vi "FaulhaberV3-Ascii_V1.vi"() -> (1 "searchnames":string[](array[string]), 2 "ID":u32[](array[numeric]), 3 "Faulhaber Objects":T3(array[cluster]))   [LabVIEW 2011] (continued)
actor\" objectType=\"7\" dataType=\"0005\" lowLimit=\"0\" highLimit=\"255\" accessType=\"rw\" defaultValue=\"0\" PDOmapping=\"no\" />\n\t\t\t\t\t<CANopenObject index=\"1010\" name=\"Store parameters\" objectType=\"8\" subNumber=\"10\">\n\t\t\t\t\t\t<CANopenSubObject subIndex=\"00\" name=\"Number of entries\" objectType=\"7\" dataType=\"0005\" accessType=\"ro\" defaultValue=\"9\" PDOmapping=\"no\" objFlags=\"0001\" />\n\t\t\t\t\t\t<CANopenSubObject subIndex=\"01\" name=\"Save all parameters\" objectType=\"7\" dataType=\"0007\" accessType=\"rw\" PDOmapping=\"no\" objFlags=\"0001\" />\n\t\t\t\t\t\t<CANopenSubObject subIndex=\"02\" name=\"Save comm parameters\" objectType=\"7\" dataType=\"0007\" accessType=\"rw\" PDOmapping=\"no\" objFlags=\"0001\" />\n\t\t\t\t\t\t<CANopenSubObject subIndex=\"03\" name=\"Save app parameters\" objectType=\"7\" dataType=\"0007\" accessType=\"rw\" PDOmapping=\"no\" objFlags=\"0001\" />\n\t\t\t\t\t\t<CANopenSubObject subIndex=\"04\" name=\"Save app parameters 1\" objectType=\"7\" dataType=\"0007\" accessType=\"rw\" PDOmapping=\"no\" objFlags=\"0003\" />\n\t\t\t\t\t\t<CANopenSubObject subIndex=\"05\" name=\"Save app parameters 2\" objectType=\"7\" dataType=\"0007\" accessType=\"rw\" PDOmapping=\"no\" objFlags=\"0003\" />\n\t\t\t\t\t\t<CANopenSubObject subIndex=\"06\" name=\"Save cal parameters\" objectType=\"7\" dataType=\"0007\" accessType=\"ro\" PDOmapping=\"no\" objFlags=\"0003\" />\n\t\t\t\t\t\t<CANopenSubObject subIndex=\"07\" name=\"Save factory parameter alls\" objectType=\"7\" dataType=\"0007\" accessType=\"ro\" PDOmapping=\"no\" objFlags=\"0003\" />\n\t\t\t\t\t\t<CANopenSubObject subIndex=\"08\" name=\"Save factory parameters com\" objectType=\"7\" dataType=\"0007\" accessType=\"ro\" PDOmapping=\"no\" objFlags=\"0003\" />\n\t\t\t\t\t\t<CANopenSubObject subIndex=\"09\" name=\"Save factory parameters app\" objectType=\"7\" dataType=\"0007\" accessType=\"ro\" PDOmapping=\"no\" objFlags=\"0003\" />\n\t\t\t\t\t</CANopenObject>\n\t\t\t\t\t<CANopenObject index=\"1011\" name=\"Restore default parameters\" objectType=\"8\" subNumber=\"7\">\n\t\t\t\t\t\t<CANopenSubObject subIndex=\"00\" name=\"Number of entries\" objectType=\"7\" dataType=\"0005\" accessType=\"ro\" defaultValue=\"6\" PDOmapping=\"no\" objFlags=\"0001\" />\n\t\t\t\t\t\t<CANopenSubObject subIndex=\"01\" name=\"Restore all default parameters\" objectType=\"7\" dataType=\"0007\" accessType=\"rw\" PDOmapping=\"no\" objFlags=\"0001\" />\n\t\t\t\t\t\t<CANopenSubObject subIndex=\"02\" name=\"Restore comm default parameters\" objectType=\"7\" dataType=\"0007\" accessType=\"rw\" PDOmapping=\"no\" objFlags=\"0001\" />\n\t\t\t\t\t\t<CANopenSubObject subIndex=\"03\" name=\"Restore app default parameters\" objectType=\"7\" dataType=\"0007\" accessType=\"rw\" PDOmapping=\"no\" objFlags=\"0001\" />\n\t\t\t\t\t\t<CANopenSubObject subIndex=\"04\" name=\"Restore app saved\" objectType=\"7\" dataType=\"0007\" accessType=\"rw\" PDOmapping=\"no\" objFlags=\"0001\" />\n\t\t\t\t\t\t<CANopenSubObject subIndex=\"05\" name=\"Restore app 1 saved\" objectType=\"7\" dataType=\"0007\" accessType=\"rw\" PDOmapping=\"no\" objFlags=\"0001\" />\n\t\t\t\t\t\t<CANopenSubObject subIndex=\"06\" name=\"Restore app 2 saved\" objectType=\"7\" dataType=\"0007\" accessType=\"rw\" PDOmapping=\"no\" objFlags=\"0001\" />\n\t\t\t\t\t</CANopenObject>\n\t\t\t\t\t<CANopenObject index=\"1014\" name=\"COB-ID EMCY\" objectType=\"7\" dataType=\"0007\" accessType=\"rw\" defaultValue=\"$NODEID+0x80\" PDOmapping=\"no\" />\n\t\t\t\t\t<CANopenObject index=\"1016\" name=\"Consumer heartbeat time\" objectType=\"8\" subNumber=\"2\">\n\t\t\t\t\t\t<CANopenSubObject subIndex=\"00\" name=\"Number of entries\" objectType=\"7\" dataType=\"0005\" accessType=\"ro\" defaultValue=\"1\" PDOmapping=\"no\" />\n\t\t\t\t\t\t<CANopenSubObject subIndex=\"01\" name=\"Consumer heartbeat time\" objectType=\"7\" dataType=\"0007\" lowLimit=\"0\" highLimit=\"0x007FFFFF\" accessType=\"rw\" defaultValue=\"0x0\" PDOmapping=\"no\" />\n\t\t\t\t\t</CANopenObject>\n\t\t\t\t\t<CANopenObject index=\"1017\" name=\"Producer heartbeat time\" objectType=\"7\" dataType=\"0006\" lowLimit=\"0\" highLimit=\"65535\" accessType=\"rw\" defaultValue=\"0\" PDOmapping=\"no\" />\n\t\t\t\t\t<CANopenObject index=\"1018\" name=\"Identity object\" objectType=\"9\" subNumber=\"5\">\n\t\t\t\t\t\t<CANopenSubObject subIndex=\"00\" name=\"Number of entries\" objectType=\"7\" dataType=\"0005\" accessType=\"ro\" defaultValue=\"4\" PDOmapping=\"no\" />\n\t\t\t\t\t\t<CANopenSubObject subIndex=\"01\" name=\"Vendor ID\" objectType=\"7\" dataType=\"0007\" accessType=\"ro\" defaultValue=\"327\" PDOmapping=\"no\" />\n\t\t\t\t\t\t<CANopenSubObject subIndex=\"02\" name=\"Product code\" objectType=\"7\" dataType=\"0007\" accessType=\"ro\" PDOmapping=\"no\" />\n\t\t\t\t\t\t<CANopenSubObject subIndex=\"03\" name=\"Revision number\" objectType=\"7\" dataType=\"0007\" lowLimit=\"0x0\" accessType=\"ro\" PDOmapping=\"no\" />\n\t\t\t\t\t\t<CANopenSubObject subIndex=\"04\" name=\"Serial number\" objectType=\"7\" dataType=\"0007\" accessType=\"ro\" PDOmapping=\"no\" />\n\t\t\t\t\t</CANopenObject>\n\t\t\t\t\t<CANopenObject index=\"1029\" name=\"Error behaviour / Number of error classes\" objectType=\"8\" subNumber=\"2\">\n\t\t\t\t\t\t<CANopenSubObject subIndex=\"00\" name=\"Number of error classes\" objectType=\"7\" dataType=\"0005\" accessType=\"ro\" defaultValue=\"1\" PDOmapping=\"no\" />\n\t\t\t\t\t\t<CANopenSubObject subIndex=\"01\" name=\"Communication error\" objectType=\"7\" dataType=\"0005\" PDOmapping=\"no\" uniqueIDRef=\"UID_PARAM_102901\" />\n\t\t\t\t\t</CANopenObject>\n\t\t\t\t\t<CANopenObject index=\"1200\" name=\"Server SDO parameter\" objectType=\"9\" subNumber=\"3\">\n\t\t\t\t\t\t<CANopenSubObject subIndex=\"00\" name=\"Number of entries\" objectType=\"7\" dataType=\"0005\" accessType=\"ro\" defaultValue=\"2\" PDOmapping=\"no\" />\n\t\t\t\t\t\t<CANopenSubObject subIndex=\"01\" name=\"COB-ID client to server (rx)\" objectType=\"7\" dataType=\"0007\" accessType=\"ro\" defaultValue=\"$NODEID+0x600\" PDOmapping=\"no\" />\n\t\t\t\t\t\t<CANopenSubObject subIndex=\"02\" name=\"COB-ID server to client (tx)\" objectType=\"7\" dataType=\"0007\" accessType=\"ro\" defaultValue=\"$NODEID+0x580\" PDOmapping=\"no\" />\n\t\t\t\t\t</CANopenObject>\n\t\t\t\t\t<CANopenObject index=\"1400\" name=\"Receive PDO1 parameter\" objectType=\"9\" subNumber=\"3\">\n\t\t\t\t\t\t<CANopenSubObject subIndex=\"00\" name=\"Number of entries\" objectType=\"7\" dataType=\"0005\" accessType=\"ro\" defaultValue=\"2\" PDOmapping=\"no\" />\n\t\t\t\t\t\t<CANopenSubObject subIndex=\"01\" name=\"COB-ID used by RxPDO1\" objectType=\"7\" dataType=\"0007\" lowLimit=\"1\" highLimit=\"4294967295\" accessType=\"rw\" defaultValue=\"$NODEID+0x200\" PDOmapping=\"no\" />\n\t\t\t\t\t\t<CANopenSubObject subIndex=\"02\" name=\"Transmission type\" objectType=\"7\" dataType=\"0005\" lowLimit=\"0\" highLimit=\"255\" accessType=\"rw\" defaultValue=\"255\" PDOmapping=\"no\" />\n\t\t\t\t\t</CANopenObject>\n\t\t\t\t\t<CANopenObject index=\"1401\" name=\"Receive PDO2 parameter\" objectType=\"9\" subNumber=\"3\">\n\t\t\t\t\t\t<CANopenSubObject subIndex=\"00\" name=\"Number of entries\" objectType=\"7\" dataType=\"0005\" accessType=\"ro\" defaultValue=\"2\" PDOmapping=\"no\" />\n\t\t\t\t\t\t<CANopenSubObject subIndex=\"01\" name=\"COB-ID used by RxPDO2\" objectType=\"7\" dataType=\"0007\" lowLimit=\"1\" highLimit=\"4294967295\" accessType=\"rw\" defaultValue=\"$NODEID+0x300\" PDOmapping=\"no\" />\n\t\t\t\t\t\t<CANopenSubObject subIndex=\"02\" name=\"Transmission type\" objectType=\"7\" dataType=\"0005\" lowLimit=\"0\" highLimit=\"255\" accessType=\"rw\" defaultValue=\"255\" PDOmapping=\"no\" />\n\t\t\t\t\t</CANopenObject>\n\t\t\t\t\t<CANopenObject index=\"1402\" name=\"Receive PDO3 parameters\" objectType=\"9\" subNumber=\"3\">\n\t\t\t\t\t\t<CANopenSubObject subIndex=\"00\" name=\"Number of entries\" objectType=\"7\" dataType=\"0005\" accessType=\"ro\" defaultValue=\"2\" PDOmapping=\"no\" />\n\t\t\t\t\t\t<CANopenSubObject subIndex=\"01\" name=\"COB-ID used by RxPDO3\" objectType=\"7\" dataType=\"0007\" lowLimit=\"1\" highLimit=\"4294967295\" accessType=\"rw\" defaultValue=\"$NODEID+0x400\" PDOmapping=\"no\" />\n\t\t\t\t\t\t<CANopenSubObject subIndex=\"02\" name=\"Transmission type\" objectType=\"7\" dataType=\"0005\" lowLimit=\"0\" highLimit=\"255\" accessType=\"rw\" defaultValue=\"255\" PDOmapping=\"no\" />\n\t\t\t\t\t</CANopenObject>\n\t\t\t\t\t<CANopenObject index=\"1403\" name=\"Receive PDO4 parameter\" objectType=\"9\" subNumber=\"3\">\n\t\t\t\t\t\t<CANopenSubObject subIndex=\"00\" name=\"Number of entries\" objectType=\"7\" dataType=\"0005\" accessType=\"ro\" defaultValue=\"2\" PDOmapping=\"no\" />\n\t\t\t\t\t\t<CANopenSubObject subIndex=\"01\" name=\"COB-ID used by RxPDO4\" objectType=\"7\" dataType=\"0007\" lowLimit=\"1\" highLimit=\"4294967295\" accessType=\"rw\" defaultValue=\"$NODEID+0x500\" PDOmapping=\"no\" />\n\t\t\t\t\t\t<CANopenSubObject subIndex=\"02\" name=\"Transmission type\" objectType=\"7\" dataType=\"0005\" lowLimit=\"0\" highLimit=\"255\" accessType=\"rw\" defaultValue=\"255\" PDOmapping=\"no\" />\n\t\t\t\t\t</CANopenObject>\n\t\t\t\t\t<CANopenObject index=\"1600\" name=\"Receive PDO1 mapping / Number of mapped objects\" objectType=\"9\" subNumber=\"5\">\n\t\t\t\t\t\t<CANopenSubObject subIndex=\"00\" name=\"Number of mapped objects\" objectType=\"7\" dataType=\"0005\" lowLimit=\"0\" highLimit=\"4\" accessType=\"rw\" defaultValue=\"1\" PDOmapping=\"no\" />\n\t\t\t\t\t\t<CANopenSubObject subIndex=\"01\" name=\"RxPDO 1 mapping entry 1\" objectType=\"7\" dataType=\"0007\" lowLimit=\"0\" highLimit=\"4294967295\" accessType=\"rw\" defaultValue=\"0x60400010\" PDOmapping=\"no\" />\n\t\t\t\t\t\t<CANopenSubObject subIndex=\"02\" name=\"RxPDO 1 Mapping entry 2\" objectType=\"7\" dataType=\"0007\" lowLimit=\"0\" highLimit=\"4294967295\" accessType=\"rw\" defaultValue=\"0x0\" PDOmapping=\"no\" />\n\t\t\t\t\t\t<CANopenSubObject subIndex=\"03\" name=\"RxPDO 1 Mapping entry 3\" objectType=\"7\" dataType=\"0007\" lowLimit=\"0\" highLimit=\"4294967295\" accessType=\"rw\" defaultValue=\"0x0\" PDOmapping=\"no\" />\n\t\t\t\t\t\t<CANopenSubObject subIndex=\"04\" name=\"RxPDO 1 Mapping entry 4\" objectType=\"7\" dataType=\"0007\" lowLimit=\"0\" highLimit=\"4294967295\" accessType=\"rw\" defaultValue=\"0x0\" PDOmapping=\"no\" />\n\t\t\t\t\t</CANopenObject>\n\t\t\t\t\t<CANopenObject index=\"1601\" name=\"Receive PDO2 mapping / Number of mapped objects\" objectType=\"9\" subNumber=\"5\">\n\t\t\t\t\t\t<CANopenSubObject subIndex=\"00\" name=\"Number of mapped objects\" objectType=\"7\" dataType=\"0005\" lowLimit=\"0\" highLimit=\"4\" accessType=\"rw\" defaultValue=\"2\" PDOmapping=\"no\" />\n\t\t\t\t\t\t<CANopenSubObject subIndex=\"01\" name=\"RxPDO2 mapping entry 1\" objectType=\"7\" dataType=\"0007\" lowLimit=\"0\" highLimit=\"4294967295\" accessType=\"rw\" defaultValue=\"0x60400010\" PDOmapping=\"no\" />\n\t\t\t\t\t\t<CANopenSubObject subIndex=\"02\" name=\"RxPDO2 mapping entry 2\" objectType=\"7\" dataType=\"0007\" lowLimit=\"0\" highLimit=\"4294967295\" accessType=\"rw\" defaultValue=\"0x607A0020\" PDOmapping=\"no\" />\n\t\t\t\t\t\t<CANopenSubObject subIndex=\"03\" name=\"RxPDO2 mapping entry 3\" objectType=\"7\" dataType=\"0007\" lowLimit=\"0\" highLimit=\"4294967295\" accessType=\"rw\" defaultValue=\"0x0\" PDOmapping=\"no\" />\n\t\t\t\t\t\t<CANopenSubObject subIndex=\"04\" name=\"RxPDO2 mapping entry 4\" objectType=\"7\" dataType=\"0007\" lowLimit=\"0\" highLimit=\"4294967295\" accessType=\"rw\" defaultValue=\"0x0\" PDOmapping=\"no\" />\n\t\t\t\t\t</CANopenObject>\n\t\t\t\t\t<CANopenObject index=\"1602\" name=\"Receive PDO3 mapping / Number of mapped objects\" objectType=\"9\" subNumber=\"5\">\n\t\t\t\t\t\t<CANopenSubObject subIndex=\"00\" name=\"Number of mapped objects\" objectType=\"7\" dataType=\"0005\" lowLimit=\"0\" highLimit=\"4\" accessType=\"rw\" defaultValue=\"2\" PDOmapping=\"no\" />\n\t\t\t\t\t\t<CANopenSubObject subIndex=\"01\" name=\"RxPDO3 mapping entry 1\" objectType=\"7\" dataType=\"0007\" lowLimit=\"0\" highLimit=\"4294967295\" accessType=\"rw\" defaultValue=\"0x60400010\" PDOmapping=\"no\" />\n\t\t\t\t\t\t<CANopenSubObject subIndex=\"02\" name=\"RxPDO3 mapping entry 2\" objectType=\"7\" dataType=\"0007\" lowLimit=\"0\" highLimit=\"4294967295\" accessType=\"rw\" defaultValue=\"0x60FF0020\" PDOmapping=\"no\" />\n\t\t\t\t\t\t<CANopenSubObject subIndex=\"03\" name=\"RxPDO3 mapping entry 3\" objectType=\"7\" dataType=\"0007\" lowLimit=\"0\" highLimit=\"4294967295\" accessType=\"rw\" defaultValue=\"0x0\" PDOmapping=\"no\" />\n\t\t\t\t\t\t<CANopenSubObject subIndex=\"04\" name=\"RxPDO3 mapping entry 4\" objectType=\"7\" dataType=\"0007\" lowLimit=\"0\" highLimit=\"4294967295\" accessType=\"rw\" defaultValue=\"0x0\" PDOmapping=\"no\" />\n\t\t\t\t\t</CANopenObject>\n\t\t\t\t\t<CANopenObject index=\"1603\" name=\"Receive PDO4 mapping / Number of mapped objects\" objectType=\"9\" subNumber=\"5\">\n\t\t\t\t\t\t<CANopenSubObject subIndex=\"00\" name=\"Number of mapped objects\" objectType=\"7\" dataType=\"0005\" lowLimit=\"0\" highLimit=\"4\" accessType=\"rw\" defaultValue=\"2\" PDOmapping=\"no\" />\n\t\t\t\t\t\t<CANopenSubObject subIndex=\"01\" name=\"RxPDO4 mapping entry 1\" objectType=\"7\" dataType=\"0007\" lowLimit=\"0\" highLimit=\"4294967295\" accessType=\"rw\" defaultValue=\"0x60400010\" PDOmapping=\"no\" />\n\t\t\t\t\t\t<CANopenSubObject subIndex=\"02\" name=\"RxPDO4 mapping entry 2\" objectType=\"7\" dataType=\"0007\" lowLimit=\"0\" highLimit=\"4294967295\" accessType=\"rw\" defaultValue=\"0x60710010\" PDOmapping=\"no\" />\n\t\t\t\t\t\t<CANopenSubObject subIndex=\"03\" name=\"RxPDO4 mapping entry 3\" objectType=\"7\" dataType=\"0007\" lowLimit=\"0\" highLimit=\"4294967295\" accessType=\"rw\" defaultValue=\"0x0\" PDOmapping=\"no\" />\n\t\t\t\t\t\t<CANopenSubObject subIndex=\"04\" name=\"RxPDO4 mapping entry 4\" objectType=\"7\" dataType=\"0007\" lowLimit=\"0\" highLimit=\"4294967295\" accessType=\"rw\" defaultValue=\"0x0\" PDOmapping=\"no\" />\n\t\t\t\t\t</CANopenObject>\n\t\t\t\t\t<CANopenObject index=\"1800\" name=\"Transmit PDO1 parameter\" objectType=\"9\" subNumber=\"4\">\n\t\t\t\t\t\t<CANopenSubObject subIndex=\"00\" name=\"Number of entries\" objectType=\"7\" dataType=\"0005\" accessType=\"ro\" defaultValue=\"5\" PDOmapping=\"no\" />\n\t\t\t\t\t\t<CANopenSubObject subIndex=\"01\" name=\"COB-ID used by TxPDO1\" objectType=\"7\" dataType=\"0007\" lowLimit=\"1\" highLimit=\"4294967295\" accessType=\"rw\" defaultValue=\"$NODEID+0x180\" PDOmapping=\"no\" />\n\t\t\t\t\t\t<CANopenSubObject subIndex=\"02\" name=\"Transmission type\" objectType=\"7\" dataType=\"0005\" lowLimit=\"0\" highLimit=\"255\" accessType=\"rw\" defaultValue=\"255\" PDOmapping=\"no\" />\n\t\t\t\t\t\t<CANopenSubObject subIndex=\"05\" name=\"Eventtimer\" objectType=\"7\" dataType=\"0006\" lowLimit=\"0\" highLimit=\"65535\" accessType=\"rw\" defaultValue=\"0\" PDOmapping=\"no\" />\n\t\t\t\t\t</CANopenObject>\n\t\t\t\t\t<CANopenObject index=\"1801\" name=\"Transmit PDO2 parameter\" objectType=\"9\" subNumber=\"4\">\n\t\t\t\t\t\t<CANopenSubObject subIndex=\"00\" name=\"Number of entries\" objectType=\"7\" dataType=\"0005\" accessType=\"ro\" defaultValue=\"5\" PDOmapping=\"no\" />\n\t\t\t\t\t\t<CANopenSubObject subIndex=\"01\" name=\"COB-ID used by TxPDO2\" objectType=\"7\" dataType=\"0007\" lowLimit=\"1\" highLimit=\"4294967295\" accessType=\"rw\" defaultValue=\"$NODEID+0x280\" PDOmapping=\"no\" />\n\t\t\t\t\t\t<CANopenSubObject subIndex=\"02\" name=\"Transmission type\" objectType=\"7\" dataType=\"0005\" lowLimit=\"0\" highLimit=\"255\" accessType=\"rw\" defaultValue=\"255\" PDOmapping=\"no\" />\n\t\t\t\t\t\t<CANopenSubObject subIndex=\"05\" name=\"Eventtimer\" objectType=\"7\" dataType=\"0006\" lowLimit=\"0\" highLimit=\"65535\" accessType=\"rw\" defaultValue=\"0\" PDOmapping=\"no\" />\n\t\t\t\t\t</CANopenObject>\n\t\t\t\t\t<CANopenObject index=\"1802\" name=\"Transmit PDO3 parameter\" objectType=\"9\" subNumber=\"4\">\n\t\t\t\t\t\t<CANopenSubObject subIndex=\"00\" name=\"Number of entries\" objectType=\"7\" dataType=\"0005\" accessType=\"ro\" defaultValue=\"5\" PDOmapping=\"no\" />\n\t\t\t\t\t\t<CANopenSubObject subIndex=\"01\" name=\"COB-ID used by TxPDO3\" objectType=\"7\" dataType=\"0007\" lowLimit=\"1\" highLimit=\"4294967295\" accessType=\"rw\" defaultValue=\"$NODEID+0x380\" PDOmapping=\"no\" />\n\t\t\t\t\t\t<CANopenSubObject subIndex=\"02\" name=\"Transmission type\" objectType=\"7\" dataType=\"0005\" lowLimit=\"0\" highLimit=\"255\" accessType=\"rw\" defaultValue=\"255\" PDOmapping=\"no\" />\n\t\t\t\t\t\t<CANopenSubObject subIndex=\"05\" name=\"Eventtimer\" objectType=\"7\" dataType=\"0006\" lowLimit=\"0\" highLimit=\"65535\" accessType=\"rw\" defaultValue=\"0\" PDOmapping=\"no\" />\n\t\t\t\t\t</CANopenObject>\n\t\t\t\t\t<CANopenObject index=\"1803\" name=\"Transmit PDO4 parameter\" objectType=\"9\" subNumber=\"4\">\n\t\t\t\t\t\t<CANopenSubObject subIndex=\"00\" name=\"Number of entries\" objectType=\"7\" dataType=\"0005\" accessType=\"ro\" defaultValue=\"5\" PDOmapping=\"no\" />\n\t\t\t\t\t\t<CANopenSubObject subIndex=\"01\" name=\"COB-ID used by TxPDO4\" objectType=\"7\" dataType=\"0007\" lowLimit=\"1\" highLimit=\"4294967295\" accessType=\"rw\" defaultValue=\"$NODEID+0x480\" PDOmapping=\"no\" />\n\t\t\t\t\t\t<CANopenSubObject subIndex=\"02\" name=\"Transmission type\" objectType=\"7\" dataType=\"0005\" lowLimit=\"0\" highLimit=\"255\" accessType=\"rw\" defaultValue=\"255\" PDOmapping=\"no\" />\n\t\t\t\t\t\t<CANopenSubObject subIndex=\"05\" name=\"Eventtimer\" objectType=\"7\" dataType=\"0006\" lowLimit=\"0\" highLimit=\"65535\" accessType=\"rw\" defaultValue=\"0\" PDOmapping=\"no\" />\n\t\t\t\t\t</CANopenObject>\n\t\t\t\t\t<CANopenObject index=\"1A00\" name=\"Transmit PDO1 mapping  / Number of mapped objects\" objectType=\"9\" subNumber=\"5\">\n\t\t\t\t\t\t<CANopenSubObject subIndex=\"00\" name=\"Number of mapped objects\" objectType=\"7\" dataType=\"0005\" lowLimit=\"0\" highLimit=\"4\" accessType=\"rw\" defaultValue=\"1\" PDOmapping=\"no\" />\n\t\t\t\t\t\t<CANopenSubObject subIndex=\"01\" name=\"TPDO1 mapping entry 1\" objectType=\"7\" dataType=\"0007\" lowLimit=\"0\" highLimit=\"4294967295\" accessType=\"rw\" defaultValue=\"0x60410010\" PDOmapping=\"no\" />\n\t\t\t\t\t\t<CANopenSubObject subIndex=\"02\" name=\"TPDO1 mapping entry 2\" objectType=\"7\" dataType=\"0007\" lowLimit=\"0\" highLimit=\"4294967295\" accessType=\"rw\" defaultValue=\"0x0\" PDOmapping=\"no\" />\n\t\t\t\t\t\t<CANopenSubObject subIndex=\"03\" name=\"TxPDO1 mapping entry 3\" objectType=\"7\" dataType=\"0007\" lowLimit=\"0\" highLimit=\"4294967295\" accessType=\"rw\" defaultValue=\"0x0\" PDOmapping=\"no\" />\n\t\t\t\t\t\t<CANopenSubObject subIndex=\"04\" name=\"TxPDO1 mapping entry 4\" objectType=\"7\" dataType=\"0007\" lowLimit=\"0\" highLimit=\"4294967295\" accessType=\"rw\" defaultValue=\"0x0\" PDOmapping=\"no\" />\n\t\t\t\t\t</CANopenObject>\n\t\t\t\t\t<CANopenObject index=\"1A01\" name=\"Transmit PDO2 mapping  / Number of mapped objects\" objectType=\"9\" subNumber=\"5\">\n\t\t\t\t\t\t<CANopenSubObject subIndex=\"00\" name=\"Number of mapped objects\" objectType=\"7\" dataType=\"0005\" lowLimit=\"0\" highLimit=\"4\" accessType=\"rw\" defaultValue=\"2\" PDOmapping=\"no\" />\n\t\t\t\t\t\t<CANopenSubObject subIndex=\"01\" name=\"TxPDO1 mapping entry 1\" objectType=\"7\" dataType=\"0007\" lowLimit=\"0\" highLimit=\"4294967295\" accessType=\"rw\" defaultValue=\"0x60410010\" PDOmapping=\"no\" />\n\t\t\t\t\t\t<CANopenSubObject subIndex=\"02\" name=\"TxPDO2 mapping entry 2\" objectType=\"7\" dataType=\"0007\" lowLimit=\"0\" highLimit=\"4294967295\" accessType=\"rw\" defaultValue=\"0x60640020\" PDOmapping=\"no\" />\n\t\t\t\t\t\t<CANopenSubObject subIndex=\"03\" name=\"TxPDO3 mapping entry 3\" objectType=\"7\" dataType=\"0007\" lowLimit=\"0\" highLimit=\"4294967295\" accessType=\"rw\" defaultValue=\"0x0\" PDOmapping=\"no\" />\n\t\t\t\t\t\t<CANopenSubObject subIndex=\"04\" name=\"TxPDO4 mapping entry 4\" objectType=\"7\" dataType=\"0007\" lowLimit=\"0\" highLimit=\"4294967295\" accessType=\"rw\" defaultValue=\"0x0\" PDOmapping=\"no\" />\n\t\t\t\t\t</CANopenObject>\n\t\t\t\t\t<CANopenObject index=\"1A02\" name=\"Transmit PDO3 mapping  / Number of mapped objects\" objectType=\"9\" subNumber=\"5\">\n\t\t\t\t\t\t<CANopenSubObject subIndex=\"00\" name=\"Number of mapped objects\" objectType=\"7\" dataType=\"0005\" lowLimit=\"0\" highLimit=\"4\" accessType=\"rw\" defaultValue=\"2\" PDOmapping=\"no\" />\n\t\t\t\t\t\t<CANopenSubObject subIndex=\"01\" name=\"TxPDO3 mapping entry 1\" objectType=\"7\" dataType=\"0007\" lowLimit=\"0\" highLimit=\"4294967295\" accessType=\"rw\" defaultValue=\"0x60410010\" PDOmapping=\"no\" />\n\t\t\t\t\t\t<CANopenSubObject subIndex=\"02\" name=\"TxPDO3 mapping entry 2\" objectType=\"7\" dataType=\"0007\" lowLimit=\"0\" highLimit=\"4294967295\" accessType=\"rw\" defaultValue=\"0x606C0020\" PDOmapping=\"no\" />\n\t\t\t\t\t\t<CANopenSubObject subIndex=\"03\" name=\"TxPDO3 mapping entry 3\" objectType=\"7\" dataType=\"0007\" lowLimit=\"0\" highLimit=\"4294967295\" accessType=\"rw\" defaultValue=\"0x0\" PDOmapping=\"no\" />\n\t\t\t\t\t\t<CANopenSubObject subIndex=\"04\" name=\"TxPDO3 mapping entry 4\" objectType=\"7\" dataType=\"0007\" lowLimit=\"0\" highLimit=\"4294967295\" accessType=\"rw\" defaultValue=\"0x0\" PDOmapping=\"no\" />\n\t\t\t\t\t</CANopenObject>\n\t\t\t\t\t<CANopenObject index=\"1A03\" name=\"Transmit PDO4 mapping  / Number of mapped objects\" objectType=\"9\" subNumber=\"5\">\n\t\t\t\t\t\t<CANopenSubObject subIndex=\"00\" name=\"Number of mapped objects\" objectType=\"7\" dataType=\"0005\" lowLimit=\"0\" highLimit=\"4\" accessType=\"rw\" defaultValue=\"2\" PDOmapping=\"no\" />\n\t\t\t\t\t\t<CANopenSubObject subIndex=\"01\" name=\"TxPDO4 mapping entry 1\" objectType=\"7\" dataType=\"0007\" lowLimit=\"0\" highLimit=\"4294967295\" accessType=\"rw\" defaultValue=\"0x60410010\" PDOmapping=\"no\" />\n\t\t\t\t\t\t<CANopenSubObject subIndex=\"02\" name=\"TxPDO4 mapping entry 2\" objectType=\"7\" dataType=\"0007\" lowLimit=\"0\" highLimit=\"4294967295\" accessType=\"rw\" defaultValue=\"0x60770010\" PDOmapping=\"no\" />\n\t\t\t\t\t\t<CANopenSubObject subIndex=\"03\" name=\"TxPDO4 mapping entry 3\" objectType=\"7\" dataType=\"0007\" lowLimit=\"0\" highLimit=\"4294967295\" accessType=\"rw\" defaultValue=\"0x0\" PDOmapping=\"no\" />\n\t\t\t\t\t\t<CANopenSubObject subIndex=\"04\" name=\"TxPDO4 mapping entry 4\" objectType=\"7\" dataType=\"0007\" lowLimit=\"0\" highLimit=\"4294967295\" accessType=\"rw\" defaultValue=\"0x0\" PDOmapping=\"no\" />\n\t\t\t\t\t</CANopenObject>\n\t\t\t\t\t<CANopenObject index=\"2300\" name=\"Number of I/Os\" objectType=\"8\" subNumber=\"5\">\n\t\t\t\t\t\t<CANopenSubObject subIndex=\"00\" name=\"Number of entries\" objectType=\"7\" dataType=\"0005\" accessType=\"ro\" defaultValue=\"4\" PDOmapping=\"no\" />\n\t\t\t\t\t\t<CANopenSubObject subIndex=\"01\" name=\"Number of digital inputs\" objectType=\"7\" dataType=\"0005\" accessType=\"ro\" PDOmapping=\"no\" objFlags=\"00020000\" />\n\t\t\t\t\t\t<CANopenSubObject subIndex=\"02\" name=\"Number of digital outputs\" objectType=\"7\" dataType=\"0005\" accessType=\"ro\" PDOmapping=\"no\" objFlags=\"00020000\" />\n\t\t\t\t\t\t<CANopenSubObject subIndex=\"03\" name=\"Number of analog inputs\" objectType=\"7\" dataType=\"0005\" accessType=\"ro\" PDOmapping=\"no\" objFlags=\"00020000\" />\n\t\t\t\t\t\t<CANopenSubObject subIndex=\"04\" name=\"Number of emulated digital inputs\" objectType=\"7\" dataType=\"0005\" PDOmapping=\"no\" objFlags=\"00020000\" uniqueIDRef=\"UID_PARAM_230004\" />\n\t\t\t\t\t</CANopenObject>\n\t\t\t\t\t<CANopenObject index=\"2310\" name=\"Digital input settings\" objectType=\"9\" subNumber=\"13\">\n\t\t\t\t\t\t<CANopenSubObject subIndex=\"00\" name=\"Number of entries\" objectType=\"7\" dataType=\"0005\" accessType=\"ro\" defaultValue=\"18\" PDOmapping=\"no\" />\n\t\t\t\t\t\t<CANopenSubObject subIndex=\"01\" name=\"Select lower limit switch inputs\" objectType=\"7\" dataType=\"0005\" PDOmapping=\"no\" objFlags=\"00020000\" uniqueIDRef=\"UID_PARAM_231001\" />\n\t\t\t\t\t\t<CANopenSubObject subIndex=\"02\" name=\"Select upper limit switch inputs\" objectType=\"7\" dataType=\"0005\" PDOmapping=\"no\" objFlags=\"00020000\" uniqueIDRef=\"UID_PARAM_231002\" />\n\t\t\t\t\t\t<CANopenSubObject subIndex=\"03\" name=\"Limit switch option code\" objectType=\"7\" dataType=\"0003\" PDOmapping=\"no\" objFlags=\"00020000\" uniqueIDRef=\"UID_PARAM_231003\" />\n\t\t\t\t\t\t<CANopenSubObject subIndex=\"04\" name=\"Select reference switch input\" objectType=\"7\" dataType=\"0005\" lowLimit=\"0\" highLimit=\"8\" accessType=\"rw\" defaultValue=\"0\" PDOmapping=\"no\" objFlags=\"00020000\" />\n\t\t\t\t\t\t<CANopenSubObject subIndex=\"05\" name=\"Emulated input threshold level\" objectType=\"7\" dataType=\"0005\" lowLimit=\"0\" highLimit=\"0x03\" accessType=\"rw\" defaultValue=\"0x00\" PDOmapping=\"no\" objFlags=\"00020000\" />\n\t\t\t\t\t\t<CANopenSubObject subIndex=\"06\" name=\"Select stop input\" objectType=\"7\" dataType=\"0005\" PDOmapping=\"no\" objFlags=\"00020000\" uniqueIDRef=\"UID_PARAM_231006\" />\n\t\t\t\t\t\t<CANopenSubObject subIndex=\"08\" name=\"Debug Write Digital Input Values\" objectType=\"7\" dataType=\"0005\" lowLimit=\"0\" highLimit=\"255\" accessType=\"wo\" PDOmapping=\"no\" objFlags=\"00020003\" />\n\t\t\t\t\t\t<CANopenSubObject subIndex=\"09\" name=\"Debug Write Brake / Fault Pin\" objectType=\"7\" dataType=\"0005\" lowLimit=\"0\" highLimit=\"255\" accessType=\"wo\" PDOmapping=\"no\" objFlags=\"00020003\" />\n\t\t\t\t\t\t<CANopenSubObject subIndex=\"0F\" name=\"Select digital inputs used\" objectType=\"7\" dataType=\"0005\" lowLimit=\"0\" highLimit=\"255\" accessType=\"rw\" defaultValue=\"0xFF\" PDOmapping=\"no\" objFlags=\"00020000\" />\n\t\t\t\t\t\t<CANopenSubObject subIndex=\"10\" name=\"Input polarity\" objectType=\"7\" dataType=\"0005\" lowLimit=\"0\" highLimit=\"255\" accessType=\"rw\" defaultValue=\"0x0\" PDOmapping=\"no\" objFlags=\"00020000\" />\n\t\t\t\t\t\t<CANopenSubObject subIndex=\"11\" name=\"Input threshold level\" objectType=\"7\" dataType=\"0005\" PDOmapping=\"no\" objFlags=\"00020000\" uniqueIDRef=\"UID_PARAM_231011\" />\n\t\t\t\t\t\t<CANopenSubObject subIndex=\"12\" name=\"Input filter active\" objectType=\"7\" dataType=\"0005\" lowLimit=\"0\" highLimit=\"255\" accessType=\"rw\" defaultValue=\"0x0\" PDOmapping=\"no\" objFlags=\"00020000\" />\n\t\t\t\t\t</CANopenObject>\n\t\t\t\t\t<CANopenObject index=\"2311\" name=\"Digital I/O status\" objectType=\"9\" subNumber=\"5\">\n\t\t\t\t\t\t<CANopenSubObject subIndex=\"00\" name=\"Number of entries\" objectType=\"7\" dataType=\"0005\" accessType=\"ro\" defaultValue=\"4\" PDOmapping=\"no\" />\n\t\t\t\t\t\t<CANopenSubObject subIndex=\"01\" name=\"Digital input logical state\" objectType=\"7\" dataType=\"0005\" lowLimit=\"0x0\" accessType=\"ro\" PDOmapping=\"TPDO\" />\n\t\t\t\t\t\t<CANopenSubObject subIndex=\"02\" name=\"Digital input physical state\" objectType=\"7\" dataType=\"0005\" lowLimit=\"0x0\" accessType=\"ro\" PDOmapping=\"TPDO\" />\n\t\t\t\t\t\t<CANopenSubObject subIndex=\"03\" name=\"Digital output status\" objectType=\"7\" dataType=\"0005\" lowLimit=\"0x0\" accessType=\"ro\" PDOmapping=\"TPDO\" objFlags=\"00020000\" />\n\t\t\t\t\t\t<CANopenSubObject subIndex=\"04\" name=\"Write digital outputs\" objectType=\"7\" dataType=\"0006\" lowLimit=\"0\" highLimit=\"65535\" accessType=\"rw\" defaultValue=\"0x0\" PDOmapping=\"RPDO\" />\n\t\t\t\t\t</CANopenObject>\n\t\t\t\t\t<CANopenObject index=\"2312\" name=\"Digital output settings\" objectType=\"9\" subNumber=\"13\">\n\t\t\t\t\t\t<CANopenSubObject subIndex=\"00\" name=\"Number of entries\" objectType=\"7\" dataType=\"0005\" accessType=\"ro\" defaultValue=\"16\" PDOmapping=\"no\" />\n\t\t\t\t\t\t<CANopenSubObject subIndex=\"01\" name=\"Select fault output pin\" objectType=\"7\" dataType=\"0005\" lowLimit=\"0\" highLimit=\"255\" accessType=\"rw\" defaultValue=\"0\" PDOmapping=\"no\" objFlags=\"00020000\" />\n\t\t\t\t\t\t<CANopenSubObject subIndex=\"02\" name=\"Select brake control pin\" objectType=\"7\" dataType=\"0005\" lowLimit=\"0\" highLimit=\"255\" accessType=\"rw\" defaultValue=\"0\" PDOmapping=\"no\" objFlags=\"00020000\" />\n\t\t\t\t\t\t<CANopenSubObject subIndex=\"03\" name=\"Brake delay time\" objectType=\"7\" dataType=\"0005\" lowLimit=\"0\" highLimit=\"255\" accessType=\"rw\" defaultValue=\"0\" PDOmapping=\"no\" objFlags=\"00020000\" />\n\t\t\t\t\t\t<CANopenSubObject subIndex=\"08\" name=\"DiagOut 1 pin selection\" objectType=\"7\" dataType=\"0005\" lowLimit=\"0\" highLimit=\"255\" accessType=\"rw\" defaultValue=\"0\" PDOmapping=\"no\" objFlags=\"00020000\" />\n\t\t\t\t\t\t<CANopenSubObject subIndex=\"09\" name=\"DiagOut 1 mask\" objectType=\"7\" dataType=\"0007\" lowLimit=\"0\" highLimit=\"4294967295\" accessType=\"rw\" defaultValue=\"0x0\" PDOmapping=\"no\" objFlags=\"00020000\" />\n\t\t\t\t\t\t<CANopenSubObject subIndex=\"0A\" name=\"DiagOut 2 pin selection\" objectType=\"7\" dataType=\"0005\" lowLimit=\"0\" highLimit=\"255\" accessType=\"rw\" defaultValue=\"0\" PDOmapping=\"no\" objFlags=\"00020000\" />\n\t\t\t\t\t\t<CANopenSubObject subIndex=\"0B\" name=\"DiagOut 2 mask\" objectType=\"7\" dataType=\"0007\" lowLimit=\"0\" highLimit=\"4294967295\" accessType=\"rw\" defaultValue=\"0x0\" PDOmapping=\"no\" objFlags=\"00020000\" />\n\t\t\t\t\t\t<CANopenSubObject subIndex=\"0C\" name=\"DiagOut 3 pin selection\" objectType=\"7\" dataType=\"0005\" lowLimit=\"0\" highLimit=\"255\" accessType=\"rw\" defaultValue=\"0\" PDOmapping=\"no\" objFlags=\"00020000\" />\n\t\t\t\t\t\t<CANopenSubObject subIndex=\"0D\" name=\"DiagOut 3 mask\" objectType=\"7\" dataType=\"0007\" lowLimit=\"0\" highLimit=\"4294967295\" accessType=\"rw\" defaultValue=\"0x0\" PDOmapping=\"no\" objFlags=\"00020000\" />\n\t\t\t\t\t\t<CANopenSubObject subIndex=\"0E\" name=\"DiagOut 4 pin selection\" objectType=\"7\" dataType=\"0005\" lowLimit=\"0\" highLimit=\"255\" accessType=\"rw\" defaultValue=\"0\" PDOmapping=\"no\" objFlags=\"00020000\" />\n\t\t\t\t\t\t<CANopenSubObject subIndex=\"0F\" name=\"DiagOut 4 mask\" objectType=\"7\" dataType=\"0007\" lowLimit=\"0\" highLimit=\"4294967295\" accessType=\"rw\" defaultValue=\"0x0\" PDOmapping=\"no\" objFlags=\"00020000\" />\n\t\t\t\t\t\t<CANopenSubObject subIndex=\"10\" name=\"Output polarity\" objectType=\"7\" dataType=\"0005\" lowLimit=\"0\" highLimit=\"0x07\" accessType=\"rw\" defaultValue=\"0x0\" PDOmapping=\"no\" objFlags=\"00020000\" />\n\t\t\t\t\t</CANopenObject>\n\t\t\t\t\t<CANopenObject index=\"2313\" name=\"Analog inputs\" objectType=\"9\" subNumber=\"21\">\n\t\t\t\t\t\t<CANopenSubObject subIndex=\"00\" name=\"Number of entries\" objectType=\"7\" dataType=\"0005\" accessType=\"ro\" defaultValue=\"26\" PDOmapping=\"no\" />\n\t\t\t\t\t\t<CANopenSubObject subIndex=\"01\" name=\"AnIn 1 gain (numerator/divisor)\" objectType=\"7\" dataType=\"0004\" lowLimit=\"-2147483648\" highLimit=\"2147483647\" accessType=\"rw\" defaultValue=\"0x7FFF8000\" PDOmapping=\"no\" objFlags=\"00020000\" />\n\t\t\t\t\t\t<CANopenSubObject subIndex=\"02\" name=\"AnIn 1 offset\" objectType=\"7\" dataType=\"0003\" lowLimit=\"-32768\" highLimit=\"32767\" accessType=\"rw\" defaultValue=\"0\" PDOmapping=\"RPDO\" objFlags=\"00020000\" />\n\t\t\t\t\t\t<CANopenSubObject subIndex=\"03\" name=\"AnIn 1 filter time\" objectType=\"7\" dataType=\"0006\" lowLimit=\"0\" highLimit=\"65535\" accessType=\"rw\" defaultValue=\"0\" PDOmapping=\"no\" objFlags=\"00020000\" />\n\t\t\t\t\t\t<CANopenSubObject subIndex=\"04\" name=\"AnIn 1 user scaled value\" objectType=\"7\" dataType=\"0004\" accessType=\"ro\" PDOmapping=\"TPDO\" objFlags=\"00020000\" />\n\t\t\t\t\t\t<CANopenSubObject subIndex=\"05\" name=\"AnIn 1 resolution as encoder\" objectType=\"7\" dataType=\"0006\" lowLimit=\"0\" highLimit=\"65535\" accessType=\"rw\" defaultValue=\"1000\" PDOmapping=\"no\" objFlags=\"00020000\" />\n\t\t\t\t\t\t<CANopenSubObject subIndex=\"06\" name=\"AnIn 1 min input limit\" objectType=\"7\" dataType=\"0003\" lowLimit=\"-32768\" highLimit=\"32767\" accessType=\"rw\" defaultValue=\"-32768\" PDOmapping=\"no\" objFlags=\"00020000\" />\n\t\t\t\t\t\t<CANopenSubObject subIndex=\"07\" name=\"AnIn 1 max input limit\" objectType=\"7\" dataType=\"0003\" lowLimit=\"-32768\" highLimit=\"32767\" accessType=\"rw\" defaultValue=\"32767\" PDOmapping=\"no\" objFlags=\"00020000\" />\n\t\t\t\t\t\t<CANopenSubObject subIndex=\"08\" name=\"AnIn 1 select dir pin\" objectType=\"7\" dataType=\"0005\" lowLimit=\"0\" highLimit=\"8\" accessType=\"rw\" defaultValue=\"0\" PDOmapping=\"no\" objFlags=\"00020000\" />\n\t\t\t\t\t\t<CANopenSubObject subIndex=\"09\" name=\"AnIn 1 virtual input value\" objectType=\"7\" dataType=\"0003\" lowLimit=\"-32768\" highLimit=\"32767\" accessType=\"rw\" defaultValue=\"0\" PDOmapping=\"RPDO\" objFlags=\"00020000\" />\n\t\t\t\t\t\t<CANopenSubObject subIndex=\"0A\" name=\"AnIn 1 enable virtual input\" objectType=\"7\" dataType=\"0005\" PDOmapping=\"RPDO\" objFlags=\"00020000\" uniqueIDRef=\"UID_PARAM_23130A\" />\n\t\t\t\t\t\t<CANopenSubObject subIndex=\"11\" name=\"AnIn 2 gain (numerator/divisor)\" objectType=\"7\" dataType=\"0004\" lowLimit=\"-2147483648\" highLimit=\"2147483647\" accessType=\"rw\" defaultValue=\"0x7FFF8000\" PDOmapping=\"no\" objFlags=\"00020000\" />\n\t\t\t\t\t\t<CANopenSubObject subIndex=\"12\" name=\"AnIn 2 offset\" objectType=\"7\" dataType=\"0003\" lowLimit=\"-32768\" highLimit=\"32767\" accessType=\"rw\" defaultValue=\"0\" PDOmapping=\"RPDO\" objFlags=\"00020000\" />\n\t\t\t\t\t\t<CANopenSubObject subIndex=\"13\" name=\"AnIn 2 filter time\" objectType=\"7\" dataType=\"0006\" lowLimit=\"0\" highLimit=\"65535\" accessType=\"rw\" defaultValue=\"0\" PDOmapping=\"no\" objFlags=\"00020000\" />\n\t\t\t\t\t\t<CANopenSubObject subIndex=\"14\" name=\"AnIn 2 user scaled value\" objectType=\"7\" dataType=\"0004\" accessType=\"ro\" PDOmapping=\"TPDO\" objFlags=\"00020000\" />\n\t\t\t\t\t\t<CANopenSubObject subIndex=\"15\" name=\"AnIn 2 resolution as encoder\" objectType=\"7\" dataType=\"0006\" lowLimit=\"0\" highLimit=\"65535\" accessType=\"rw\" defaultValue=\"1000\" PDOmapping=\"no\" objFlags=\"00020000\" />\n\t\t\t\t\t\t<CANopenSubObject subIndex=\"16\" name=\"AnIn 2 min input limit\" objectType=\"7\" dataType=\"0003\" lowLimit=\"-32768\" highLimit=\"32767\" accessType=\"rw\" defaultValue=\"-32768\" PDOmapping=\"no\" objFlags=\"00020000\" />\n\t\t\t\t\t\t<CANopenSubObject subIndex=\"17\" name=\"AnIn 2 max input limit\" objectType=\"7\" dataType=\"0003\" lowLimit=\"-32768\" highLimit=\"32767\" accessType=\"rw\" defaultValue=\"32767\" PDOmapping=\"no\" objFlags=\"00020000\" />\n\t\t\t\t\t\t<CANopenSubObject subIndex=\"18\" name=\"AnIn 2 select dir pin\" objectType=\"7\" dataType=\"0005\" lowLimit=\"0\" highLimit=\"8\" accessType=\"rw\" defaultValue=\"0\" PDOmapping=\"no\" objFlags=\"00020000\" />\n\t\t\t\t\t\t<CANopenSubObject subIndex=\"19\" name=\"AnIn 2 virtual input value\" objectType=\"7\" dataType=\"0003\" lowLimit=\"-32768\" highLimit=\"32767\" accessType=\"rw\" defaultValue=\"0\" PDOmapping=\"RPDO\" objFlags=\"00020000\" />\n\t\t\t\t\t\t<CANopenSubObject subIndex=\"1A\" name=\"AnIn 2 enable virtual input\" objectType=\"7\" dataType=\"0005\" PDOmapping=\"RPDO\" objFlags=\"00020000\" uniqueIDRef=\"UID_PARAM_23131A\" />\n\t\t\t\t\t</CANopenObject>\n\t\t\t\t\t<CANopenObject index=\"2314\" name=\"Manufacturer scaled analog input values\" objectType=\"8\" subNumber=\"13\">\n\t\t\t\t\t\t<CANopenSubObject subIndex=\"00\" name=\"Number of entries\" objectType=\"7\" dataType=\"0005\" accessType=\"ro\" defaultValue=\"12\" PDOmapping=\"no\" />\n\t\t\t\t\t\t<CANopenSubObject subIndex=\"01\" name=\"AnIn 1 scaled value (IA)\" objectType=\"7\" dataType=\"0003\" accessType=\"ro\" PDOmapping=\"TPDO\" />\n\t\t\t\t\t\t<CANopenSubObject subIndex=\"02\" name=\"AnIn 2 scaled value (IB)\" objectType=\"7\" dataType=\"0003\" accessType=\"ro\" PDOmapping=\"TPDO\" />\n\t\t\t\t\t\t<CANopenSubObject subIndex=\"03\" name=\"AnIn 3 scaled value (IC)\" objectType=\"7\" dataType=\"0003\" accessType=\"ro\" PDOmapping=\"TPDO\" />\n\t\t\t\t\t\t<CANopenSubObject subIndex=\"04\" name=\"AnIn 4 scaled value (Hall A)\" objectType=\"7\" dataType=\"0003\" accessType=\"ro\" PDOmapping=\"TPDO\" />\n\t\t\t\t\t\t<CANopenSubObject subIndex=\"05\" name=\"AnIn 5 scaled value (Hall B)\" objectType=\"7\" dataType=\"0003\" accessType=\"ro\" PDOmapping=\"TPDO\" />\n\t\t\t\t\t\t<CANopenSubObject subIndex=\"06\" name=\"AnIn 6 scaled value (Hall C)\" objectType=\"7\" dataType=\"0003\" accessType=\"ro\" PDOmapping=\"TPDO\" />\n\t\t\t\t\t\t<CANopenSubObject subIndex=\"07\" name=\"AnIn 7 scaled value \" objectType=\"7\" dataType=\"0003\" accessType=\"ro\" PDOmapping=\"TPDO\" />\n\t\t\t\t\t\t<CANopenSubObject subIndex=\"08\" name=\"AnIn 8 scaled value \" objectType=\"7\" dataType=\"0003\" accessType=\"ro\" PDOmapping=\"TPDO\" />\n\t\t\t\t\t\t<CANopenSubObject subIndex=\"09\" name=\"AnIn 9 scaled value \" objectType=\"7\" dataType=\"0003\" accessType=\"ro\" PDOmapping=\"TPDO\" />\n\t\t\t\t\t\t<CANopenSubObject subIndex=\"0A\" name=\"AnIn 10 scaled value \" objectType=\"7\" dataType=\"0003\" accessType=\"ro\" PDOmapping=\"TPDO\" />\n\t\t\t\t\t\t<CANopenSubObject subIndex=\"0B\" name=\"AnIn 11 scaled value \" objectType=\"7\" dataType=\"0003\" accessType=\"ro\" PDOmapping=\"TPDO\" />\n\t\t\t\t\t\t<CANopenSubObject subIndex=\"0C\" name=\"AnIn 12 scaled value \" objectType=\"7\" dataType=\"0003\" accessType=\"ro\" PDOmapping=\"TPDO\" />\n\t\t\t\t\t</CANopenObject>\n\t\t\t\t\t<CANopenObject index=\"2315\" name=\"Motor encoder\" objectType=\"9\" subNumber=\"11\">\n\t\t\t\t\t\t<CANopenSubObject subIndex=\"00\" name=\"Number of entries\" objectType=\"7\" dataType=\"0005\" accessType=\"ro\" defaultValue=\"10\" PDOmapping=\"no\" />\n\t\t\t\t\t\t<CANopenSubObject subIndex=\"01\" name=\"Operation mode, index polarity\" objectType=\"7\" dataType=\"0006\" lowLimit=\"0\" highLimit=\"0x9F07\" accessType=\"rw\" defaultValue=\"0x0\" PDOmapping=\"no\" objFlags=\"00020000\" />\n\t\t\t\t\t\t<CANopenSubObject subIndex=\"02\" name=\"IE resolution\" objectType=\"7\" dataType=\"0007\" lowLimit=\"0\" highLimit=\"4194304\" accessType=\"rw\" PDOmapping=\"no\" objFlags=\"00020000\" />\n\t\t\t\t\t\t<CANopenSubObject subIndex=\"03\" name=\"Motor encoder position\" objectType=\"7\" dataType=\"0004\" accessType=\"ro\" PDOmapping=\"TPDO\" />\n\t\t\t\t\t\t<CANopenSubObject subIndex=\"04\" name=\"Gain  (numerator/divisor)\" objectType=\"7\" dataType=\"0004\" lowLimit=\"-2147483648\" highLimit=\"2147483647\" accessType=\"rw\" defaultValue=\"0x40004000\" PDOmapping=\"RPDO\" objFlags=\"00020000\" />\n\t\t\t\t\t\t<CANopenSubObject subIndex=\"05\" name=\"MotorEnc scaled position\" objectType=\"7\" dataType=\"0004\" lowLimit=\"-2147483648\" highLimit=\"2147483647\" accessType=\"rw\" PDOmapping=\"TPDO\" />\n\t\t\t\t\t\t<CANopenSubObject subIndex=\"06\" name=\"Absolute encoder bits\" objectType=\"7\" dataType=\"0007\" lowLimit=\"0x0\" highLimit=\"4294967295\" accessType=\"rw\" PDOmapping=\"no\" objFlags=\"00020000\" />\n\t\t\t\t\t\t<CANopenSubObject subIndex=\"07\" name=\"Encoder status\" objectType=\"7\" dataType=\"0005\" accessType=\"ro\" defaultValue=\"0\" PDOmapping=\"TPDO\" objFlags=\"00020000\" />\n\t\t\t\t\t\t<CANopenSubObject subIndex=\"08\" name=\"Motor encoder act speed\" objectType=\"7\" dataType=\"0004\" accessType=\"ro\" PDOmapping=\"TPDO\" />\n\t\t\t\t\t\t<CANopenSubObject subIndex=\"09\" name=\"Speed filter\" objectType=\"7\" dataType=\"0006\" lowLimit=\"0\" highLimit=\"65535\" accessType=\"rw\" defaultValue=\"10\" PDOmapping=\"TPDO\" objFlags=\"00020000\" />\n\t\t\t\t\t\t<CANopenSubObject subIndex=\"0A\" name=\"Single turn position 16 bit\" objectType=\"
